vi "LV2 Global.vi"(0 "Home Ref In":refnum<vi>, 5 "Mode Ref In":refnum<vi>, 7 "Configuration Ref In":refnum<vi>, 9 "Status Ref In":refnum<vi>, 11 "Error In":errorcluster, 13 "Enum":T1) -> (4 "Home Ref":refnum<vi>, 6 "Mode Ref":refnum<vi>, 8 "Configuration Ref":refnum<vi>, 10 "Status Ref":refnum<vi>, 15 "Error Out":errorcluster)   [LabVIEW 2020, in "INL DNL Test.lvclass"]
doc: "LV2 to write and read the asynchronously called VI"
uses:
  INL DNL Test.lvclass
  Parent/Typedef/LV2 Control.ctl
  Parent/Test.lvclass
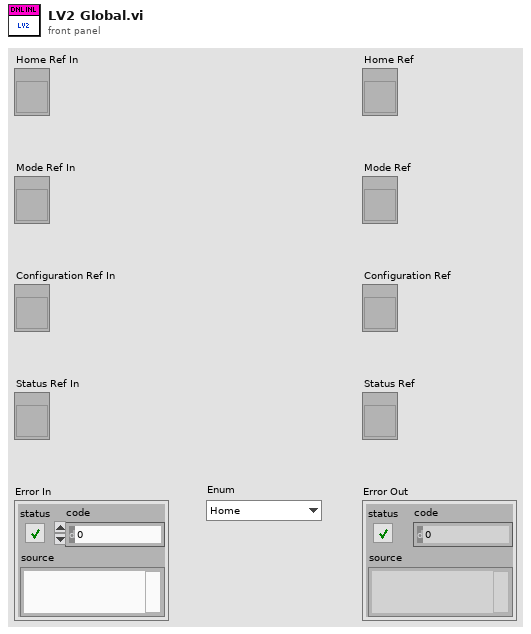
[diagram p1: front panel]
types:
  T1 = typedef "Test.lvclass/LV2 Control.ctl" = enum16{"Home", "Mode", "Config", "Status", "Read"}
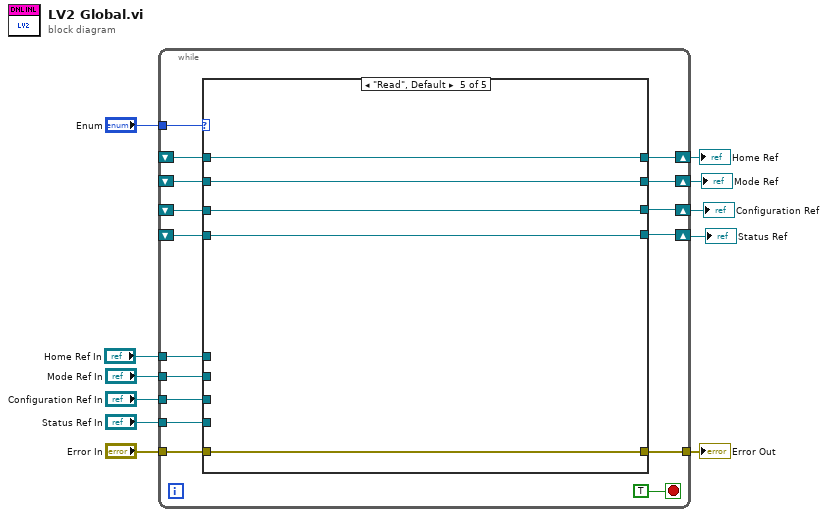
[diagram p0: block diagram]
diagram:
  n1 = while {
    tunnel: "Enum" -> [w27]
    tunnel: "Error In" -> [w25]
    tunnel: [w24] -> w9
    tunnel: "Home Ref In" -> [w23]
    shift-right: [w22] -> w1
    shift-left: _ -> [w21]
    tunnel: "Mode Ref In" -> [w20]
    shift-right: [w19] -> w7
    shift-left: _ -> [w18]
    tunnel: "Configuration Ref In" -> [w17]
    shift-right: [w16] -> w5
    shift-left: _ -> [w15]
    tunnel: "Status Ref In" -> [w14]
    shift-right: [w13] -> w3
    shift-left: _ -> [w12]
    stop <- TRUE stop-if-true
    n2 = case shown="\"Read\", Default" w27 {
      tunnel: w25 -> [w32 w33 w38 w43 w52]
      tunnel: [w32 w33 w38 w43 w52] -> w24
      tunnel: w23 -> [w31 _ _ _ _]
      tunnel: [w31 w37 w42 w47 w51] -> w22
      tunnel: w21 -> [_ w37 w42 w47 w51]
      tunnel: w20 -> [_ w34 _ _ _]
      tunnel: [w30 w34 w39 w46 w50] -> w19
      tunnel: w18 -> [w30 _ w39 w46 w50]
      tunnel: w17 -> [_ _ w41 _ _]
      tunnel: [w29 w36 w41 w45 w49] -> w16
      tunnel: w15 -> [w29 w36 _ w45 w49]
      tunnel: w14 -> [_ _ _ w44 _]
      tunnel: [w28 w35 w40 w44 w48] -> w13
      tunnel: w12 -> [w28 w35 w40 _ w48]
      frame "Home" {
      }
      frame "Mode" {
      }
      frame "Config" {
      }
      frame "Status" {
      }
      frame "Read", Default {
      }
    }
  }
  "Error Out" <- w9
  "Mode Ref" <- w7
  "Configuration Ref" <- w5
  "Status Ref" <- w3
  "Home Ref" <- w1
